vi "Connect.vi"(8 "Error In":errorcluster, 10 "Resource Name":refnum<k15>, 11 "object in":refnum<class "IStates.lvclass">) -> (0 "Error Out":errorcluster, 2 "Resource Name out":refnum<k15>, 3 "object out":refnum<class "IStates.lvclass">)   [LabVIEW 2023, in "HAL.lvlib" / "FGEN.lvlib" / "IStates.lvclass"]
uses:
  IStates.lvclass
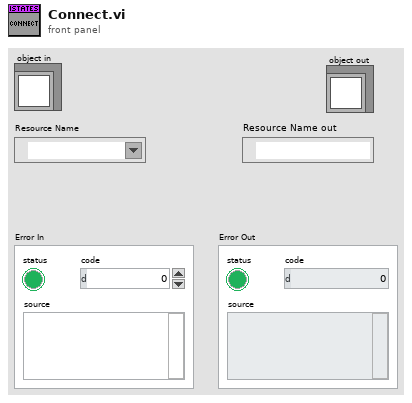
[diagram p1: front panel]
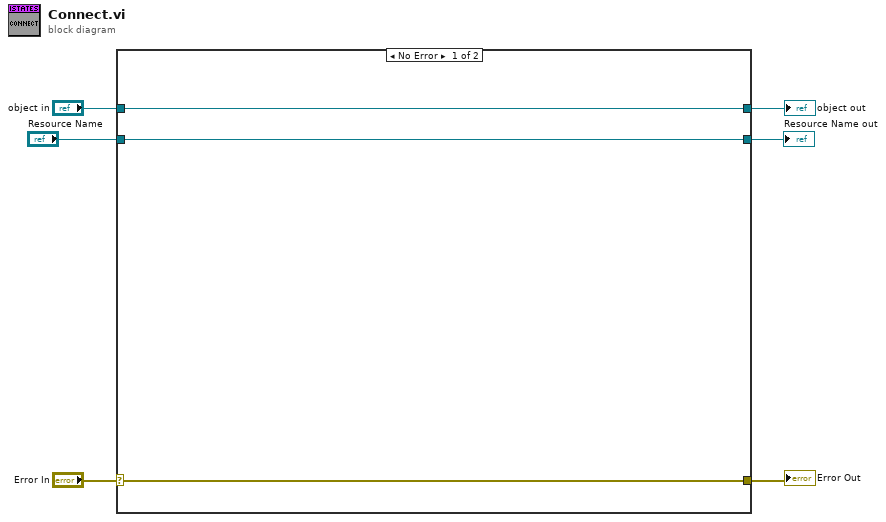
[diagram p0: block diagram]
diagram:
  n1 = case shown="No Error" "Error In" {
    selector: "Error In" -> [w9 w12]
    tunnel: [w9 w12] -> w5
    tunnel: [w8 w11] -> w3
    tunnel: "object in" -> [w8 w11]
    tunnel: "Resource Name" -> [w7 w10]
    tunnel: [w7 w10] -> w1
    frame No Error {
    }
    frame Error {
    }
  }
  "Error Out" <- w5
  "object out" <- w3
  "Resource Name out" <- w1
